vi "waveform deconvolution.vi"(7 "ignore timestamp?":bool, 8 "error in (no error)":errorcluster, 10 "kernel":waveform(dbl)={"t0"=timestamp(0 s since 1904-01-01), "dt"=0.0, "Y"=[]}, 11 "convolved signal":waveform(dbl)={"t0"=timestamp(0 s since 1904-01-01), "dt"=0.0, "Y"=[]}) -> (0 "error out":errorcluster, 3 "original signal":waveform(dbl))   [LabVIEW 2020, in "NI_MAPro.lvlib"]
uses:
  NI_MAPro.lvlib
  NI_AALPro.lvlib
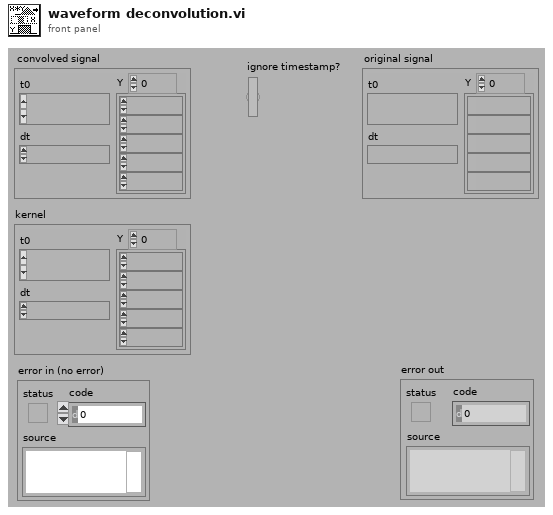
[diagram p1: front panel]
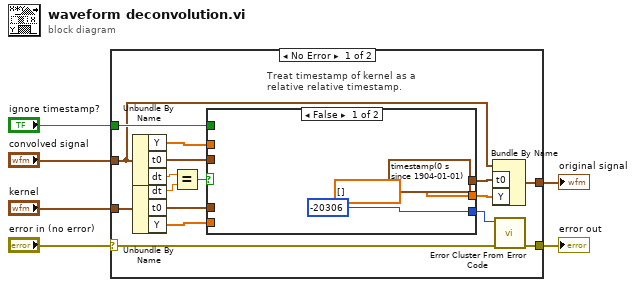
[diagram p0: block diagram]
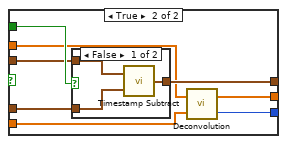
[diagram p2: hidden frame]
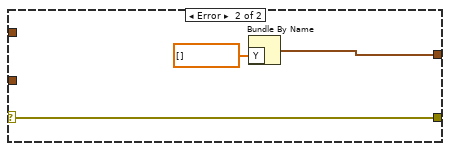
[diagram p4: hidden frame]
diagram:
  n1 = case shown="No Error" "error in (no error)" {
    selector: "error in (no error)" -> [w11 w40]
    tunnel: "convolved signal" -> [w8 _]
    tunnel: "kernel" -> [w21 _]
    tunnel: [w7 w39] -> w4
    tunnel: [w12 w40] -> w2
    tunnel: "ignore timestamp?" -> [w22 _]
    frame No Error {
      # "Treat timestamp of kernel as a \nrelative relative timestamp."
      n2 = Unbundle By Name(w8) -> ("Y"=w20:dbl[], "t0"=w16:timestamp, "dt"=w19:dbl)
      n3 = Unbundle By Name(w21) -> ("dt"=w14:dbl, "t0"=w15:timestamp, "Y"=w18:dbl[])
      n4 = Equal?(x=w19, y=w14) -> (x = y?=w17:bool)
      n5 = case shown="False" w17 {
        tunnel: w20 -> [_ w27]
        tunnel: w18 -> [_ w32]
        tunnel: w16 -> [_ w31]
        tunnel: w15 -> [_ w30]
        tunnel: [-20306 w29] -> w13
        tunnel: [timestamp(0 s since 1904-01-01) w28] -> w10
        tunnel: [dbl[] [] ("X * Y") w26] -> w9
        tunnel: w22 -> [_ w33]
        frame False {
        }
        frame True {
          n6 = case shown="False" w33 {
            tunnel: w31 -> [w36 w37]
            tunnel: w30 -> [w35 _]
            tunnel: [w34 w37] -> w28
            frame False {
              n7 = call "Timestamp Subtract.vi"("y"=w35, "x"=w36) -> ("x - y"=w34:timestamp)
            }
            frame True {
            }
          }
          n8 = call "Deconvolution.vi"("Y"=w32, "X * Y"=w27) -> ("error"=w29:i32, "X"=w26:dbl[])
        }
      }
      n9 = Bundle By Name(cluster=w8, "t0"=w10, "Y"=w9) -> (w7:waveform(dbl))
      n10 = call "Error Cluster From Error Code.vi"("error in (no error)"=w11, "error code (0)"=w13) -> ("error out"=w12:errorcluster)  [unwired: 7 in]
    }
    frame Error {
      n11 = Bundle By Name("Y"=dbl[] []) -> (w39:waveform(dbl))  [unwired: 1 in]
    }
  }
  "original signal" <- w4
  "error out" <- w2
